vi "Add Entry.vi"(5 "BG Color (None)":u32(colorbox), 6 "Parent (None)":string[](array[string]), 7 "Name Prefix (none)":string, 8 "error in":errorcluster, 9 "Columns":string[](array[string]), 10 "Name":string, 11 "Tree Map in":refnum<class "Project Tree Map.lvclass">) -> (0 "error out":errorcluster, 3 "Tree Map out":refnum<class "Project Tree Map.lvclass">, 4 "Hierarchy":string[](array[string]))   [LabVIEW 2020, in "Project Tree.lvlib" / "Project Tree Map.lvclass"]
uses:
  Project Tree Map.lvclass
  Project Tree Map.lvclass/Project Tree Map.ctl
  Tree Entry.ctl
  Tree Key.ctl
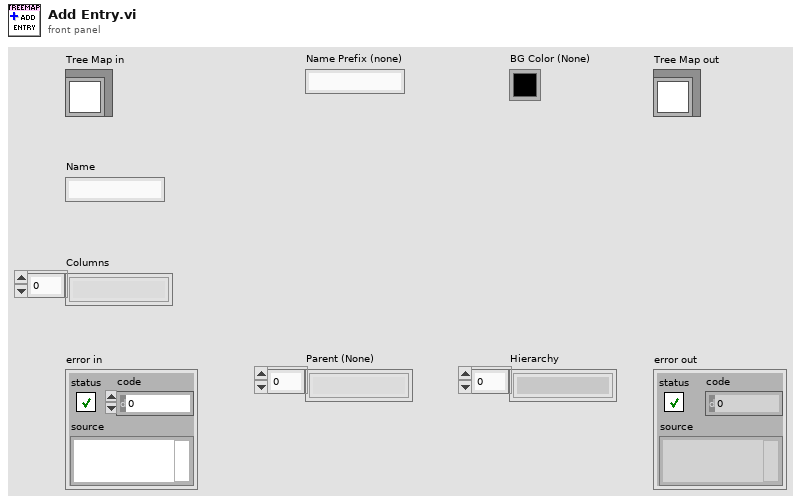
[diagram p1: front panel]
types:
  T1 = typedef "Project Tree.lvlib/Project Tree Map.lvclass/Tree Entry.ctl" = cluster{"Hierarchy":string[], "Name":string, "Columns":string[], "BG Color":u32, "Leaf":bool, "Symbol":string}
  T2 = typedef "imagedata.ctl" = cluster{"image type":i32, "image depth":i32, "image":u8[], "mask":u8[], "colors":u32[], "Rectangle":cluster{"left":i16, "top":i16, "right":i16, "bottom":i16}}
  T3 = map{string, cluster{"index":i32, "image data":T2}}
  T4 = typedef "Project Tree.lvlib/Project Tree Map.lvclass/Tree Key.ctl" = cluster{"Order":i32, "Hierarchy":string[]}
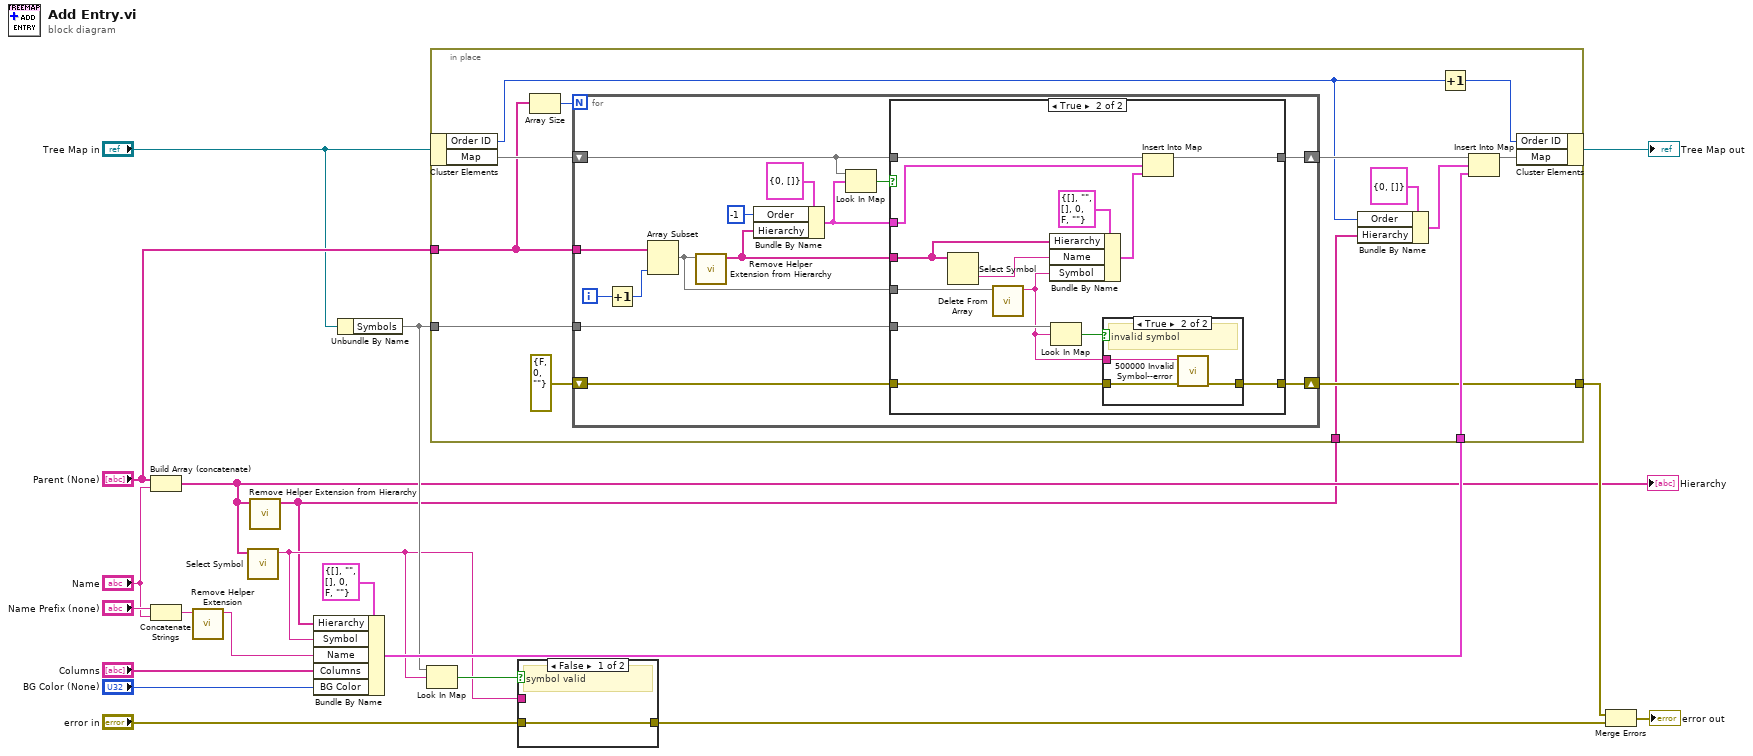
[diagram p0: block diagram]
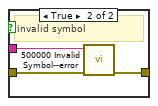
[diagram p4: hidden frame]
diagram:
  n1 = Build Array (concatenate)("Parent (None)", "Name") -> (w3:string[])
  "Hierarchy" <- w3
  n2 = Concatenate Strings("Name Prefix (none)", "Name") -> (w5:string)
  n3 = call "Remove Helper Extension.vi"("Filename"=w5) -> ("Filename without Helper Extension"=w4:string)  [unwired: 10 in]
  n4 = call "Select Symbol.vi"("Hierarchy"=w3) -> ("Symbol ID"=w2:string)  [unwired: 10 in]
  n5 = call "Remove Helper Extension from Hierarchy.vi"("Hierarchy"=w3) -> ("Hierarchy without Helper Extensions"=w1:string[])  [unwired: 10 in]
  n6 = Bundle By Name(cluster=T1 {"Hierarchy"=[], "Name"="", "Columns"=[], "BG Color"=0, "Leaf"=FALSE, "Symbol"=""} ("Tree Entry"), "Hierarchy"=w1, "Symbol"=w2, "Name"=w4, "Columns"="Columns", "BG Color"="BG Color (None)") -> (w13:T1)
  n7 = Unbundle By Name("Tree Map in") -> ("Symbols"=w8:T3)
  n8 = Look In Map(map=w8, key=w2) -> (key not found?=w6:bool)  [unwired: 1 in, 1 out]
  n9 = in-place {
    in-place-border: w13 -> [w34]
    in-place-border: w1 -> [w24]
    in-place-border: "Parent (None)" -> [w30]
    in-place-border: [w28] -> w9
    in-place-border: w8 -> [w27]
    n10 = in-place-cluster #1("Tree Map in") -> ("Order ID"=w22:i32, "Map"=w32:map{T4, T1})
    n11 = Array Size(array=w30) -> (size(s)=w29:i32)
    n12 = for {
      N: w29 -> [_]
      shift-right: [w44] -> w31
      shift-left: w32 -> [w45]
      tunnel: w30 -> [w48]
      tunnel: w27 -> [w41]
      shift-right: [w42] -> w28
      shift-left: errorcluster {"status"=FALSE, "code"=0, "source"=""} ("error out") -> [w40]
      i -> [w47]
      n13 = Increment(x=w47) -> (x+1=w43:i32)
      n14 = Array Subset(array=w48, length=w43) -> (w39:string[])  [unwired: 1 in]
      n15 = call "Remove Helper Extension from Hierarchy.vi"("Hierarchy"=w39) -> ("Hierarchy without Helper Extensions"=w35:string[])  [unwired: 10 in]
      n16 = Bundle By Name(cluster=T4 {"Order"=0, "Hierarchy"=[]} ("key"), "Order"=-1, "Hierarchy"=w35) -> (w36:T4)
      n17 = Look In Map(map=w45, key=w36) -> (key not found?=w46:bool)  [unwired: 1 in, 1 out]
      n18 = case shown="True" w46 {
        tunnel: w45 -> [w50 w63]
        tunnel: w35 -> [_ w54]
        tunnel: [w50 w62] -> w44
        tunnel: [w49 w57] -> w42
        tunnel: w41 -> [_ w59]
        tunnel: w40 -> [w49 w56]
        tunnel: w39 -> [_ w52]
        tunnel: w36 -> [_ w51]
        frame False {
        }
        frame True {
          n19 = Delete From Array(array=w54) -> (deleted portion=w53:string)  [unwired: 2 in, 1 out]
          n20 = call "Select Symbol.vi"("Hierarchy"=w52) -> ("Symbol ID"=w55:string)  [unwired: 10 in]
          n21 = Bundle By Name(cluster=T1 {"Hierarchy"=[], "Name"="", "Columns"=[], "BG Color"=0, "Leaf"=FALSE, "Symbol"=""} ("value"), "Hierarchy"=w54, "Name"=w53, "Symbol"=w55) -> (w60:T1)
          n22 = Look In Map(map=w59, key=w55) -> (key not found?=w58:bool)  [unwired: 1 in, 1 out]
          n23 = case shown="True" w58 {
            tunnel: [w64 w67] -> w57
            tunnel: w55 -> [_ w66]
            tunnel: w56 -> [w64 w65]
            frame False {
              # "symbol valid"
            }
            frame True {
              # "invalid symbol"
              n24 = call "500000 Invalid Symbol--error.vi"("error in"=w65, "Argument"=w66) -> ("error out"=w67:errorcluster)  [unwired: 8 in, 1 out]
            }
          }
          n25 = Insert Into Map(map in=w63, key=w51, value=w60) -> (map out=w62:map{T4, T1})  [unwired: 2 out]
        }
      }
    }
    n26 = Bundle By Name(cluster=T4 {"Order"=0, "Hierarchy"=[]} ("key"), "Order"=w22, "Hierarchy"=w24) -> (w23:T4)
    n27 = Increment(x=w22) -> (x+1=w21:i32)
    n28 = Insert Into Map(map in=w31, key=w23, value=w34) -> (map out=w33:map{T4, T1})  [unwired: 2 out]
    n29 = in-place-cluster #1("Order ID"=w21, "Map"=w33) -> (→"Tree Map out":refnum<class "Project Tree Map.lvclass">)
  }
  n30 = case shown="False" w6 {
    tunnel: "error in" -> [w68 w71]
    tunnel: [w68 w70] -> w12
    tunnel: w2 -> [_ w69]
    frame False {
      # "symbol valid"
    }
    frame True {
      # "invalid symbol"
      n31 = call "500000 Invalid Symbol--error.vi"("error in"=w71, "Argument"=w69) -> ("error out"=w70:errorcluster)  [unwired: 8 in, 1 out]
    }
  }
  n32 = Merge Errors(w9, w12) -> (→"error out":errorcluster)
